vi "Kd报文计算公式.vi"(1 "Kd":dbl(slide) scale=0.0..5.0 scale format="%#_4g") -> (0 "Kd报文":string)   [LabVIEW 2023]
panel:
  out "输出字符串":string
  in  "选项卡控件":enum32{"选项卡 1", "选项卡 2"}(tab)
  out "十进制数":i32
  out "16进制字符串":string
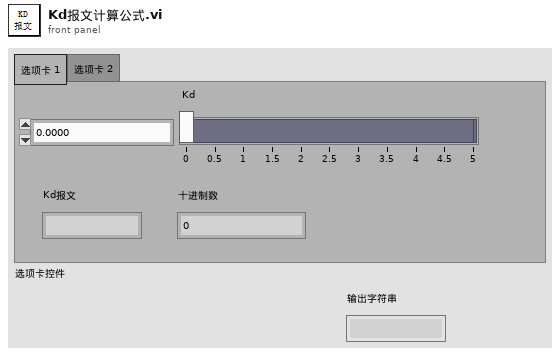
[diagram p1: front panel]
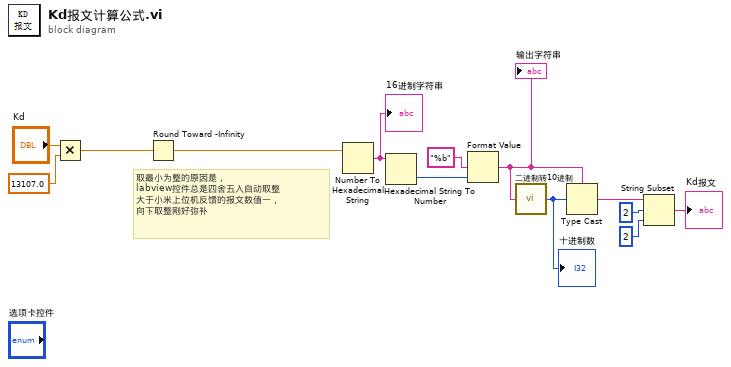
[diagram p0: block diagram]
diagram:
  # "取最小为整的原因是，\nlabview控件总是四舍五入自动取整\n大于小米上位机反馈的报文数值一，\n向下取整刚好弥补"
  n1 = Multiply(x="Kd", y=13107.0) -> (x*y=w4:dbl)
  n2 = Round Toward -Infinity(1:w4) -> (0:w3:dbl)
  n3 = Number To Hexadecimal String(2:w3) -> (0:w10:string)  [unwired: 1 in]
  "16进制字符串" <- w10
  n4 = Hexadecimal String To Number(string=w10) -> (number=w2:u32)  [unwired: 2 in, 1 out]
  n5 = Format Value(format string="%b" ("格式字符串"), value (0)=w2) -> (output string=w1:string)  [unwired: 1 in]
  "输出字符串" <- w1
  n6 = call "二进制转10进制.vi"("字符串"=w1) -> ("十进制数"=w11:i32)
  "十进制数" <- w11
  n7 = Type Cast(type=w1, x=w11) -> (*(type *) &x=w9:string)
  n8 = String Subset(string=w9, offset (0)=2 ("偏移量(0)"), length (rest)=2 ("长度（剩余）")) -> (substring=→"Kd报文":string)
